vi "Revision Query.vi"(8 "error in (no error)":errorcluster, 11 "VISA resource name":refnum<visa-resource-name>) -> (0 "error out":errorcluster, 1 "Main Firmware Revision":string, 2 "Boot Firmware Revision":string, 3 "VISA resource name out":refnum<visa-resource-name>, 5 "Instrument Driver Revision":string)   [LabVIEW 2015, in "JY-SPEX-TRIAX.lvlib"]
doc: "Queries the current instrument firmware revision and instrument driver revision (for both the boot and main firmware)."
uses:
  JY-SPEX-TRIAX.lvlib
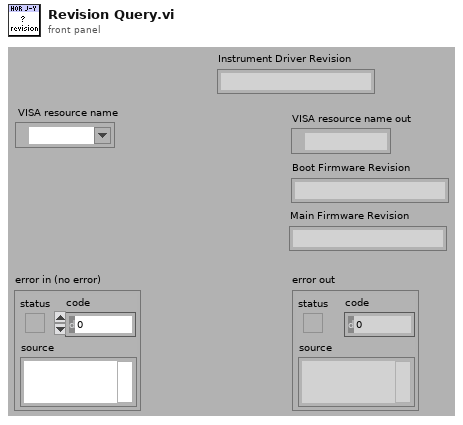
[diagram p1: front panel]
types:
  T1 = enum32{"invalid app kind", "Development System", "Run Time System", "Student Edition", "Embedded LabVIEW", "Evaluation", "Custom"}
  T2 = cluster{"Major":u16, "Minor":u16, "Fix":u16, "Build":u16}
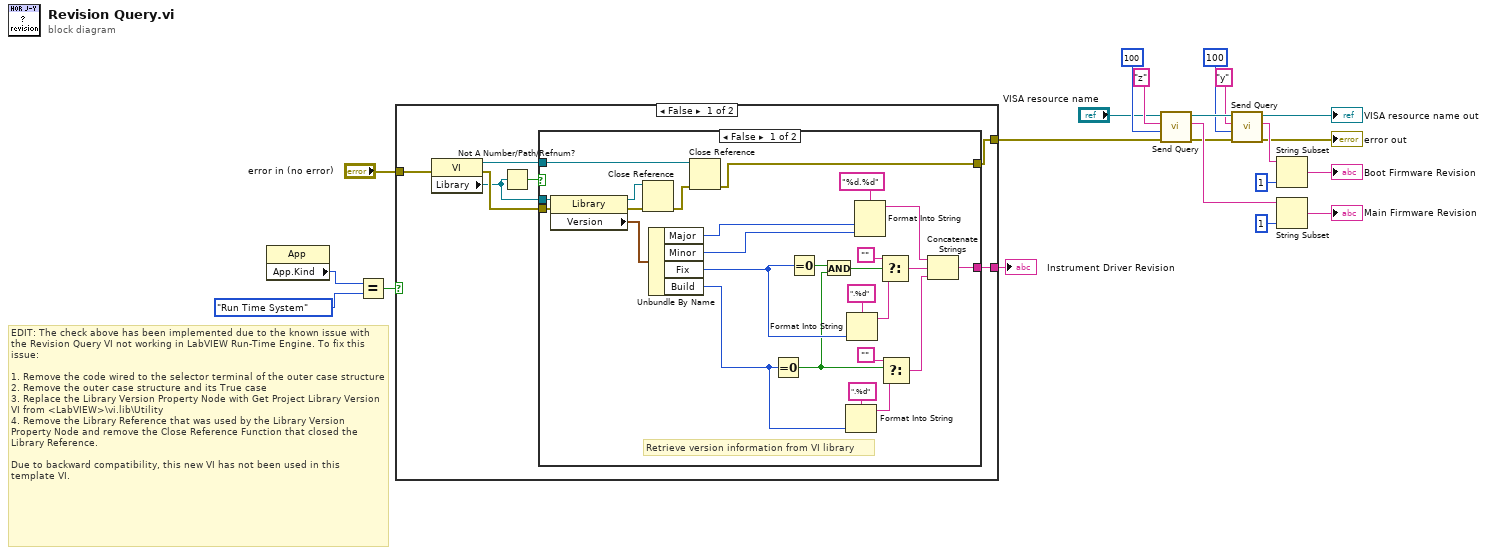
[diagram p0: block diagram]
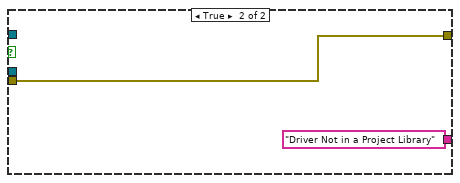
[diagram p2: hidden frame]
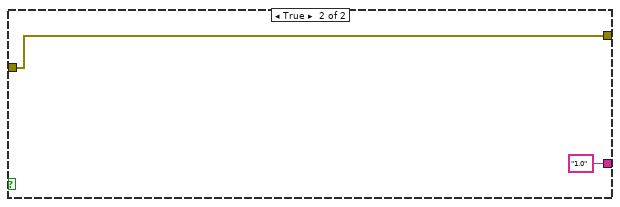
[diagram p3: hidden frame]
diagram:
  # "EDIT: The check above has been implemented due to the known issue with the Revision Query VI not working in LabVIEW Run-Time Engine. To fix this issue:\n\n1. Remove the code wired to the selector terminal of the outer case structure\n2. Remove the outer case structure and its True case\n3. Replace the Library Version Property Node with Get Project Library Version VI from <LabVIEW>\\vi.lib\\Utility\n4. Remove the Library Reference that was used by the Library Version Property Node and remove the Close Reference Function that closed the Library Reference.\n\nDue to backward compatibility, this new VI has not been used in this template VI."
  n1 = property class="App"() -> ("App.Kind"=w18:T1)  [unwired: 2 in, 2 out]
  n2 = Equal?(x=w18, y=T1."Run Time System" ("Application:Kind")) -> (x = y?=w19:bool)
  n3 = case shown="False" w19 {
    tunnel: [w24 "1.0"] -> w21
    tunnel: "error in (no error)" -> [w23 w57]
    tunnel: [w22 w57] -> w13
    frame False {
      n4 = property class="VI"(error in=w23) -> (reference out=w28:refnum<vi>, error out=w27:errorcluster, "Library"=w26:refnum<vi>)  [unwired: 1 in]
      n5 = Not A Number/Path/Refnum?(number/path/refnum=w26) -> (NaN/Path/Refnum?=w25:bool)
      n6 = case shown="False" w25 {
        tunnel: w28 -> [w51 _]
        tunnel: w27 -> [w36 w56]
        tunnel: [w31 w56] -> w22
        tunnel: [w30 "Driver Not in a Project Library"] -> w24
        tunnel: w26 -> [w29 _]
        frame False {
          # "Retrieve version information from VI library"
          n7 = property class="Library"(reference=w29, error in=w36) -> (reference out=w53:refnum<vi>, error out=w54:errorcluster, "Version"=w50:T2)
          n8 = Close Reference(reference=w53, error in (no error)=w54) -> (error out=w52:errorcluster)
          n9 = Unbundle By Name(w50) -> ("Major"=w39:u16, "Minor"=w38:u16, "Fix"=w35:u16, "Build"=w37:u16)
          n10 = Close Reference(reference=w51, error in (no error)=w52) -> (error out=w31:errorcluster)
          n11 = Equal To 0?(x=w37) -> (x = 0?=w33:bool)
          n12 = Equal To 0?(x=w35) -> (x = 0?=w34:bool)
          n13 = And(x=w34, y=w33) -> (x .and. y?=w32:bool)
          n14 = Format Into String(format string=".%d", w37) -> (resulting string=w43:string)  [unwired: 2 in, 1 out]
          n15 = Format Into String(format string=".%d", w35) -> (resulting string=w47:string)  [unwired: 2 in, 1 out]
          n16 = Format Into String(format string="%d.%d", w39, w38) -> (resulting string=w45:string)  [unwired: 2 in, 1 out]
          n17 = Select(t="", s=w32, f=w47) -> (s? t:f=w44:string)
          n18 = Select(t="", s=w33, f=w43) -> (s? t:f=w40:string)
          n19 = Concatenate Strings(w45, w44, w40) -> (w30:string)
        }
        frame True {
        }
      }
    }
    frame True {
    }
  }
  "Instrument Driver Revision" <- w21
  n20 = call "Send Query.vi"("error in (no error)"=w13, "byte count"=u32 100 ("Bytes to Read"), "write buffer"="z" ("Revision Query Command"), "VISA resource name"="VISA resource name") -> ("error out"=w9:errorcluster, "read buffer"=w12:string, "VISA resource name out"=w10:refnum<visa-resource-name>)  [unwired: 5 out]
  n21 = call "Send Query.vi"("error in (no error)"=w9, "byte count"=u32 100, "write buffer"="y", "VISA resource name"=w10) -> ("error out"=→"error out":errorcluster, "read buffer"=w7:string, "VISA resource name out"=→"VISA resource name out":refnum<visa-resource-name>)  [unwired: 5 out]
  n22 = String Subset(string=w7, offset (0)=1) -> (substring=→"Boot Firmware Revision":string)  [unwired: 1 out]
  n23 = String Subset(string=w12, offset (0)=1) -> (substring=→"Main Firmware Revision":string)  [unwired: 1 out]
